vi "sv_Append Virtual Reference_Copy.vi"(6 "SV Signal in":refnum<class "SV Signal.lvclass">, 7 "reset":bool, 8 "error in (no error)":errorcluster, 11 "acquired waveforms":waveform(dbl)[](array[waveform])) -> (0 "error out":errorcluster, 3 "acquired waveforms with virtual reference":waveform(dbl)[](array[waveform]))   [LabVIEW 2021, in "Audio ADC Shared.lvlib"]
uses:
  <vilib>/addons/_NISVFA/_Generation/Signal Generation/SV Signal/SV Signal.lvclass
  <vilib>/addons/_NISVFA/_Shared subVIs/Controls/NI Channel Properties.ctl
  <vilib>/addons/_NISVFA/_Generation/Signal Generation/SV Signal/Read Sample Rate.vi
  <vilib>/measure/maresamp.llb/Resample Waveform (single shot).vi
  Audio ADC Shared.lvlib
  <vilib>/measure/NI_MAPro.lvlib
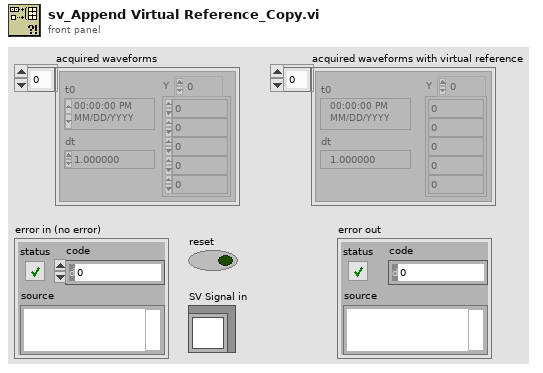
[diagram p1: front panel]
types:
  T1 = typedef "NI Channel Properties.ctl" = u16
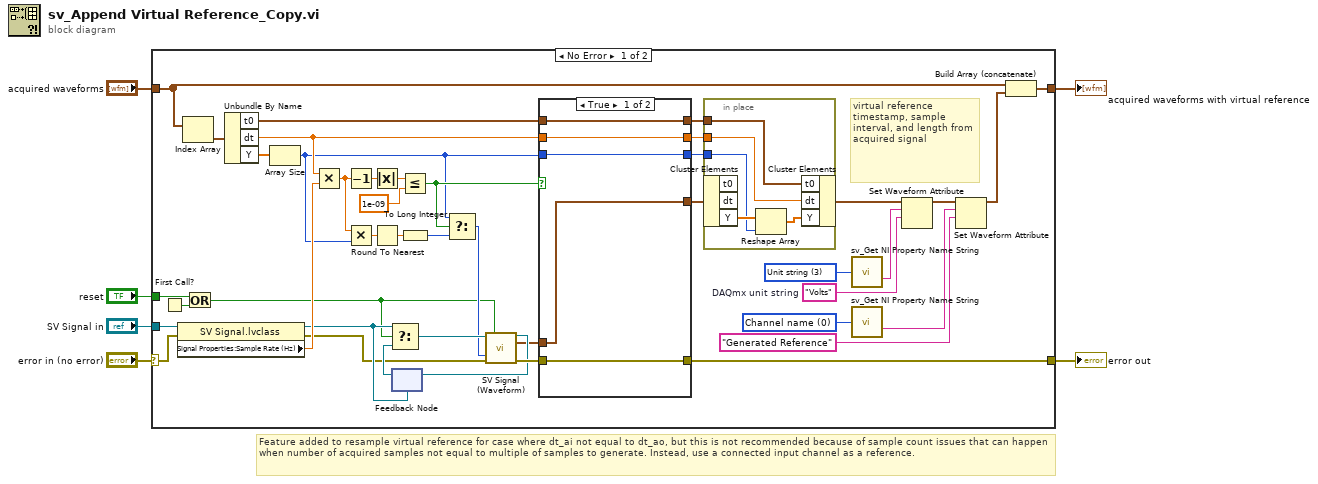
[diagram p0: block diagram]
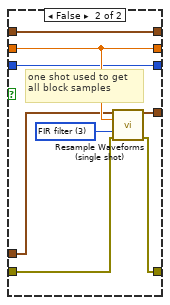
[diagram p2: hidden frame]
diagram:
  # "Feature added to resample virtual reference for case where dt_ai not equal to dt_ao, but this is not recommended because of sample count issues that can happen when number of acquired samples not equal to multiple of samples to generate. Instead, use a connected input channel as a reference."
  n1 = case shown="No Error" "error in (no error)" {
    selector: "error in (no error)" -> [w39 w68]
    tunnel: "acquired waveforms" -> [w48 w69]
    tunnel: [w47 w69] -> w5
    tunnel: [w18 w68] -> w4
    tunnel: "SV Signal in" -> [w40 _]
    tunnel: "reset" -> [w42 _]
    frame No Error {
      w24 = T1 0 items=["Channel name", "Channel description", "Axis label", "Unit string", "Waveform X-axis label", "Waveform X-axis unit string", "x0", "dx", "Number of samples", "X channel", "Filter settled", "dB reference", "Window", "Window parameter", "Window size", "FFT size", "Peak units", "Spectrum type", "Magnitude scale", "Spectral density", "Sensor sensitivity (mV/EU)", "X-axis dimension", "LabVIEW datatype", "Function type", "Function subtype", "X values", "Independent channel", "Column index", "Collection name", "Collection ID", "X Columns", "Phase unwrapped", "Sensor type", "Sensor maximum", "Averaging mode"] ("property")
      w21 = "Volts"  # DAQmx unit string
      w23 = T1 3 items=["Channel name", "Channel description", "Axis label", "Unit string", "Waveform X-axis label", "Waveform X-axis unit string", "x0", "dx", "Number of samples", "X channel", "Filter settled", "dB reference", "Window", "Window parameter", "Window size", "FFT size", "Peak units", "Spectrum type", "Magnitude scale", "Spectral density", "Sensor sensitivity (mV/EU)", "X-axis dimension", "LabVIEW datatype", "Function type", "Function subtype", "X values", "Independent channel", "Column index", "Collection name", "Collection ID", "X Columns", "Phase unwrapped", "Sensor type", "Sensor maximum", "Averaging mode"] ("property")
      # "virtual reference timestamp, sample interval, and length from acquired signal"
      n2 = First Call?() -> (First Call?: T/F=w43:bool)
      n3 = property on="Property Node" class="SV Signal.lvclass"(reference=w40, error in=w39) -> (reference out=w32:refnum<class "SV Signal.lvclass">, error out=w14:errorcluster, "Signal Properties:Sample Rate (Hz)"=w34:dbl)
      n4 = Index Array(array=w48) -> (element=w44:waveform(dbl))  [unwired: 1 in]
      n5 = Or(x=w42, y=w43) -> (x .or. y?=w11:bool)
      n6 = Unbundle By Name ("Get Waveform Components")(w44) -> ("t0"=w45:timestamp, "dt"=w38:dbl, "Y"=w49:dbl[])
      n7 = Array Size(array=w49) -> (size(s)=w7:i32)
      n8 = Multiply(x=w38, y=w34) -> (x*y=w31:dbl)
      n9 = Decrement(x=w31) -> (x-1=w37:dbl)
      n10 = Multiply(x=w31, y=w7) -> (x*y=w30:dbl)
      n11 = Absolute Value(x=w37) -> (abs(x)=w36:dbl)
      n12 = Round To Nearest(number=w30) -> (nearest integer value=w29:dbl)
      n13 = feedback #1(w32) -> (w33:refnum<class "SV Signal.lvclass">)
      n14 = Select(t=w32, s=w11, f=w33) -> (s? t:f=w15:refnum<class "SV Signal.lvclass">)
      n15 = Less Or Equal?(x=w36, y=1e-09) -> (x <= y?=w17:bool)
      n16 = To Long Integer(number=w29) -> (32bit integer=w16:i32)
      n17 = Select(t=w7, s=w17, f=w16) -> (s? t:f=w12:i32)
      n18 = call-dynamic "SV Signal (Waveform).vi"("signal configuration"=w15, "reset"=w11, "samples"=w12, "error in (no error)"=w14) -> ("signal configuration"=w10:refnum<class "SV Signal.lvclass">, "output waveform"=w9:waveform(dbl), "error out"=w13:errorcluster)  [unwired: 6 in, 3 out]
      n19 = feedback-in #1(w10) -> ()
      n20 = case shown="True" w17 {
        tunnel: w45 -> [w59 w65]
        tunnel: [w57 w63] -> w18
        tunnel: w13 -> [w57 w62]
        tunnel: w38 -> [w58 w66]
        tunnel: [w56 w64] -> w25
        tunnel: [w58 w66] -> w27
        tunnel: [w59 w65] -> w26
        tunnel: w9 -> [w56 w61]
        tunnel: [w55 w60] -> w8
        tunnel: w7 -> [w55 w60]
        frame True {
        }
        frame False {
          w67 = u16 3 items=["coerce", "linear", "spline", "FIR filter"] ("interpolation mode")
          # "one shot used to get all block samples"
          n21 = call-poly <vilib>:"Resample Waveforms (single shot).vi"("waveform in"=w61, "dt"=w66, "interpolation mode"=w67, "error in (no error)"=w62) -> ("resampled waveform out"=w64:waveform(dbl), "error out"=w63:errorcluster)  [unwired: 8 in, 2 out]
        }
      }
      n22 = in-place "In Place Element Structure" {
        in-place-border: w26 -> [w54]
        in-place-border: w27 -> [w53]
        in-place-border: w8 -> [w51]
        n23 = in-place-cluster #2(w25) -> ("Y"=w52:dbl[])  [unwired: 2 out]
        n24 = Reshape Array(w52, w51) -> (w50:dbl[])
        n25 = in-place-cluster #2("t0"=w54, "dt"=w53, "Y"=w50) -> (w28:waveform(dbl))
      }
      n26 = call <vilib>:"sv_Get NI Property Name String.vi"("property"=w23) -> ("WDT attribute name"=w20:string)  [unwired: 13 in, 1 out]
      n27 = call <vilib>:"sv_Get NI Property Name String.vi"("property"=w24) -> ("WDT attribute name"=w22:string)  [unwired: 13 in, 1 out]
      n28 = Set Waveform Attribute(5:w21, 6:w20, 7:w28) -> (3:w41:waveform(dbl))  [unwired: 1 in, 2 out]
      n29 = Set Waveform Attribute(5:"Generated Reference" ("name"), 6:w22, 7:w41) -> (3:w46:waveform(dbl))  [unwired: 1 in, 2 out]
      n30 = Build Array (concatenate)(w48, w46) -> (w47:waveform(dbl)[])
    }
    frame Error {
    }
  }
  "acquired waveforms with virtual reference" <- w5
  "error out" <- w4
